vi "two_button_change.vi"(5 "lower limit":u8, 6 "Unit of change":u8, 7 "upper limit":u8, 9 "Position in":u8, 10 "Decrement":bool, 11 "Increment":bool) -> (2 "Position out":u8, 3 "Update?":bool)   [LabVIEW 2012, in "Serenity_mk2.lvrbt"]
uses:
  Serenity_mk2.lvrbt
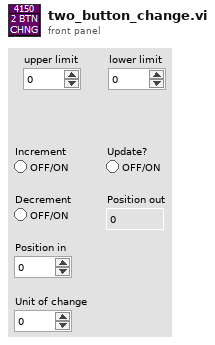
[diagram p1: front panel]
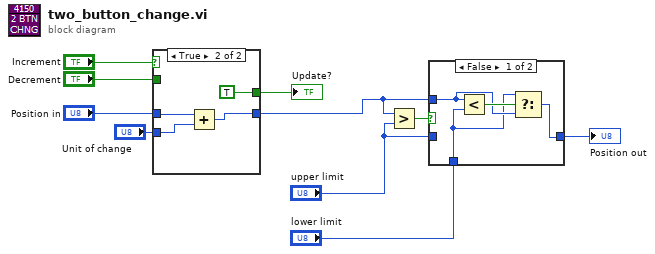
[diagram p0: block diagram]
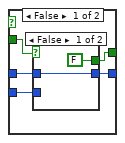
[diagram p3: hidden frame]
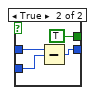
[diagram p4: hidden frame]
diagram:
  n1 = case shown="True" "Increment" {
    tunnel: "Decrement" -> [w15 _]
    tunnel: "Position in" -> [w14 w25]
    tunnel: [w13 w24] -> w3
    tunnel: [w12 TRUE] -> w9
    tunnel: "Unit of change" -> [w11 w22]
    frame False {
      n2 = case shown="False" w15 {
        tunnel: w14 -> [w17 w21]
        tunnel: [w17 w20] -> w13
        tunnel: [FALSE TRUE] -> w12
        tunnel: w11 -> [_ w18]
        frame False {
        }
        frame True {
          n3 = Subtract(x=w21, y=w18) -> (x-y=w20:u8)
        }
      }
    }
    frame True {
      n4 = Add(x=w25, y=w22) -> (x+y=w24:u8)
    }
  }
  "Update?" <- w9
  n5 = Greater?(x=w3, y="upper limit") -> (0:w5:bool)
  n6 = case shown="False" w5 {
    tunnel: "upper limit" -> [_ w30]
    tunnel: [w26 w30] -> w1
    tunnel: w3 -> [w28 _]
    tunnel: "lower limit" -> [w27 _]
    frame False {
      n7 = Less?(x=w28, y=w27) -> (x < y?=w29:bool)
      n8 = Select(t=w27, s=w29, f=w28) -> (s? t:f=w26:u8)
    }
    frame True {
    }
  }
  "Position out" <- w1
